vi "Digital PPMU Measure.vi"(7 "milliseconds to wait":u32, 8 "Published Data Id":string[](array[string]), 9 "measurement type":T1=2401 items=["Voltage"=2401, "Current"=2400], 10 "Pin Names":string[](array[string]), 11 "Semiconductor Module Context":T2) -> (0 "error out":errorcluster)   [LabVIEW 2014]
uses:
  <vilib>/NI_TestStand_SemiconductorModule/NI_TestStand_Semiconductor_Module.lvlibp/PinMap/General/SemiconductorModuleContext.ctl
  <instrlib>/niDigital/niDigital.llb/niDigital Measurement Type.ctl
  <vilib>/NI_TestStand_SemiconductorModule/NI_TestStand_Semiconductor_Module.lvlibp/PinMap/Digital Pattern/PinsToNIDigitalPatternSessions.vi
  <vilib>/NI_TestStand_SemiconductorModule/NI_TestStand_Semiconductor_Module.lvlibp/PinMap/General/Publish/PublishDataDoubleFunctionalTest.vi
  <vilib>/NI_TestStand_SemiconductorModule/NI_TestStand_Semiconductor_Module.lvlibp
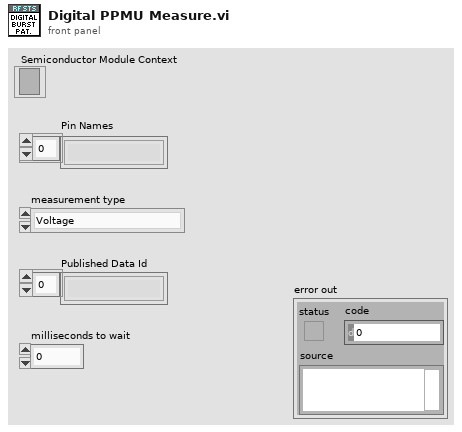
[diagram p1: front panel]
types:
  T1 = typedef "niDigital Measurement Type.ctl" = i32
  T2 = typedef "NI_TestStand_Semiconductor_Module.lvlibp/SemiconductorModuleContext.ctl" = refnum<k7>
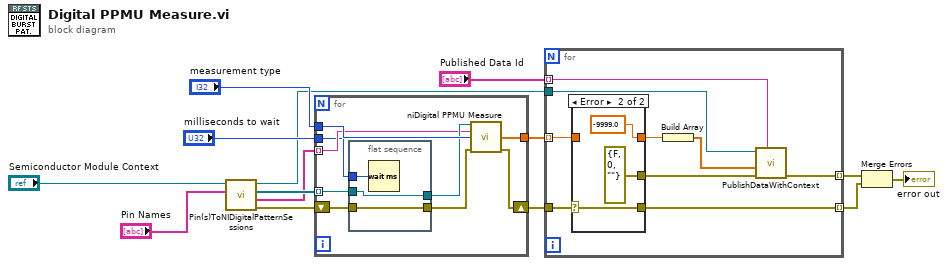
[diagram p0: block diagram]
diagram:
  n1 = call-poly <vilib>:"Pin(s)ToNIDigitalPatternSessions.vi"("Pins"="Pin Names", "Semiconductor Module Context"="Semiconductor Module Context") -> ("error out"=w8:errorcluster, "Channel Lists"=w11:string[], "Instrument Sessions"=w12:refnum<k15>[], "Semiconductor Module Context Out"=w7:T2)  [unwired: 4 in, 2 out]
  n2 = for {
    tunnel: w12 -> [w16] mode=indexing
    tunnel: w11 -> [w19] mode=indexing
    tunnel: [w22] -> w5
    tunnel: "measurement type" -> [w21]
    tunnel: "milliseconds to wait" -> [w17]
    shift-right: [w23] -> w6
    shift-left: w8 -> [w15]
    n3 = flat-sequence {
      tunnel: [w26] -> w20
      tunnel: w16 -> [w26]
      tunnel: w15 -> [w25]
      tunnel: [w25] -> w18
      tunnel: w17 -> [w24]
      frame #0 {
        n4 = Wait (ms)(milliseconds to wait=w24) -> ()  [unwired: 1 out]
      }
    }
    n5 = call <instrlib>:"niDigital PPMU Measure.vi"("instrument handle"=w20, "channel list"=w19, "measurement type"=w21, "error in"=w18) -> ("measurements"=w22:dbl[], "error out"=w23:errorcluster)  [unwired: 9 in, 1 out]
  }
  n6 = for {
    tunnel: w7 -> [w35]
    tunnel: w5 -> [w31] mode=indexing
    tunnel: "Published Data Id" -> [w33] mode=indexing
    tunnel: w6 -> [w30]
    tunnel: [w34] -> w3 mode=indexing
    tunnel: [w27] -> w2 mode=indexing
    n7 = case shown="Error" w30 {
      selector: w30 -> [w36 w39]
      tunnel: w31 -> [w37 _]
      tunnel: [w37 -9999.0 ("detected fundamental\nfrequency [Hz]")] -> w29
      tunnel: [w36 errorcluster {"status"=FALSE, "code"=0, "source"=""} ("error IO")] -> w28
      tunnel: [w36 w39] -> w27
      frame No Error {
      }
      frame Error {
      }
    }
    n8 = Build Array(w29) -> (w32:dbl[])
    n9 = call-poly <vilib>:"PublishDataWithContext.vi"("Published Data Id"=w33, "error in (no error)"=w28, "Data In"=w32, "Semiconductor Module Context"=w35) -> ("error out"=w34:errorcluster)  [unwired: 6 in, 1 out]
  }
  n10 = Merge Errors(w3, w2) -> (→"error out":errorcluster)
